vi "Write WorkDir.vi"(8 "error in (no error)":errorcluster, 10 "Work Dir":path, 11 "HIJ Vision Application in":refnum<class "HIJ Vision Application.lvclass">) -> (0 "error out":errorcluster, 3 "HIJ Vision Application out":refnum<class "HIJ Vision Application.lvclass">)   [LabVIEW 2020, in "HIJ Vision Application.lvlib" / "HIJ Vision Application.lvclass"]
uses:
  HIJ Vision Application.lvclass
  HIJ Vision Application.lvclass/HIJ Vision Application.ctl
  Display Actors/HIJ Vision Display/HIJ Vision Display Messages/Write WorkDir Msg/Write WorkDir Msg.lvclass/Write WorkDir Msg.ctl
  <vilib>/ActorFramework/Message Enqueuer/Message Enqueuer.lvclass/Message Enqueuer.ctl
  Read Display Enq.vi
  <vilib>/ActorFramework/Message Enqueuer/Enqueue.vi
  Display Actors/HIJ Vision Display/HIJ Vision Display Messages/Write WorkDir Msg/Write WorkDir Msg.lvclass
  C:/Program Files (x86)/National Instruments/LabVIEW 2020/vi.lib/ActorFramework/Message/Message.lvclass
  <vilib>/ActorFramework/Message Priority Queue/Priority Enqueue.vi
  <vilib>/ActorFramework/Message Enqueuer/Message Enqueuer.lvclass
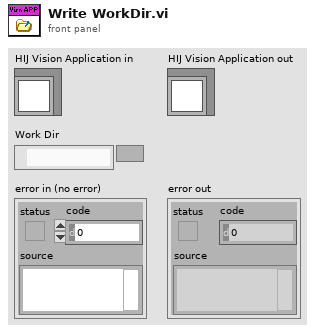
[diagram p1: front panel]
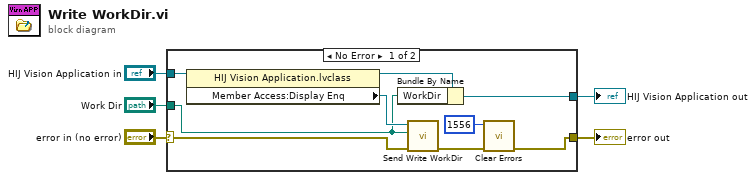
[diagram p0: block diagram]
diagram:
  n1 = case shown="No Error" "error in (no error)" {
    selector: "error in (no error)" -> [w11 w16]
    tunnel: [w7 w16] -> w4
    tunnel: [w9 w15] -> w2
    tunnel: "HIJ Vision Application in" -> [w14 w15]
    tunnel: "Work Dir" -> [w8 _]
    frame No Error {
      n2 = property class="HIJ Vision Application.lvclass"(reference=w14) -> (reference out=w13:refnum<class "HIJ Vision Application.lvclass">, "Member Access:Display Enq"=w12:refnum<class "Message Enqueuer.lvclass">)  [unwired: 1 in, 1 out]
      n3 = Bundle By Name(cluster=w13, "WorkDir"=w8) -> (w9:refnum<class "HIJ Vision Application.lvclass">)
      n4 = call "Send Write WorkDir.vi"("error in (no error)"=w11, "WorkDir"=w8, "Message Enqueuer"=w12) -> ("error out"=w10:errorcluster)  [unwired: 7 in, 1 out]
      n5 = call <vilib>:"Clear Errors.vi"("error in (no error)"=w10, "specific error code to clear (0: all)"=1556) -> ("error out"=w7:errorcluster)  [unwired: 4 in, 1 out]
    }
    frame Error {
    }
  }
  "error out" <- w4
  "HIJ Vision Application out" <- w2
